vi "VI Tree.vi"   [LabVIEW 2020, in "Rohde&Schwarz CMXP Base.lvlib"]
doc: "This is the instrument driver for the Rohde&Schwarz CMX/CMP/PVT Base system. \n\nThe VI Tree displays all the user-callable VIs of the instrument driver in an organized table.\n\nFor detailed driver information including modification history, refer to the <B>rsvna.chm </B>file."
uses:
  <instrlib>/Rohde&Schwarz CMXP Base/Rohde&Schwarz CMXP Base.lvlib
panel:
  # "rsCmxpBase"
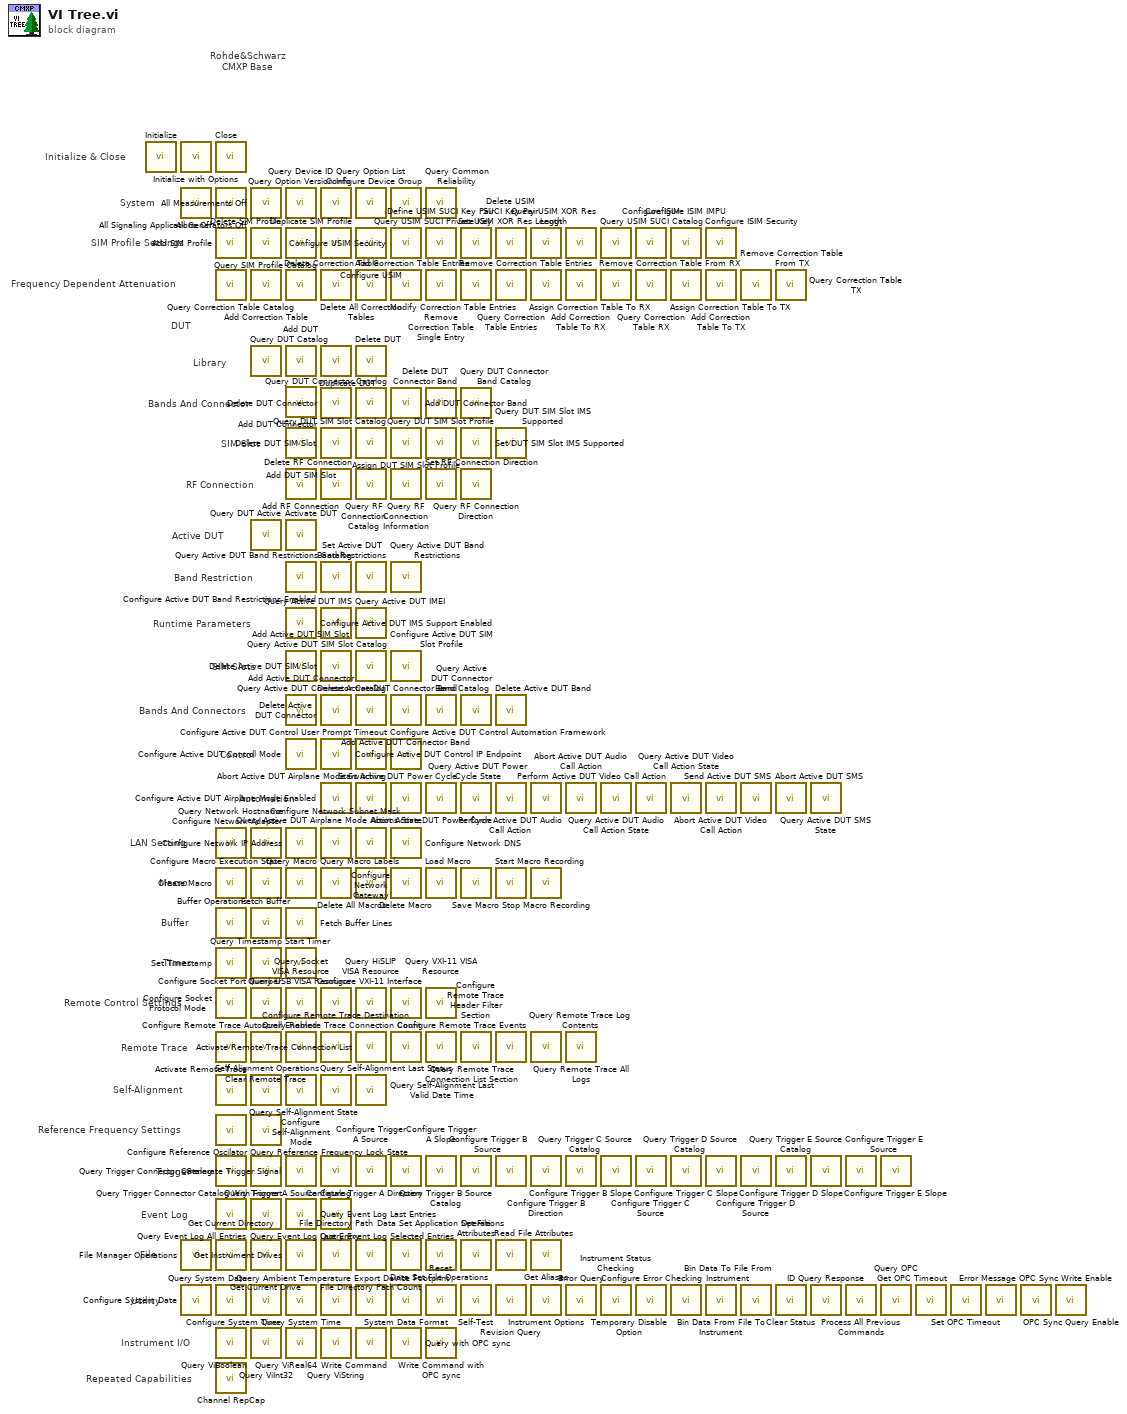
[diagram p0: block diagram]
diagram:
  # "Repeated Capabilities"
  # "Automation"
  # "Control"
  # "Bands And Connectors"
  # "SIM Slots"
  # "Runtime Parameters"
  # "Band Restriction"
  # "RF Connection"
  # "Active DUT"
  # "SIM Slot"
  # "Bands And Connector"
  # "Library"
  # "DUT"
  # "Frequency Dependent Attenuation"
  # "Remote Trace"
  # "Event Log"
  # "Trigger"
  # "File"
  # "Reference Frequency Settings"
  # "Self-Alignment"
  # "Remote Control Settings"
  # "Timer"
  # "Buffer"
  # "Macro"
  # "LAN Setting"
  # "SIM Profile Settings"
  # "System"
  # "Rohde&Schwarz \n    CMXP Base"
  # "Instrument I/O"
  # "Utility"
  # "Initialize & Close"
  n1 = call <instrlib>:"Initialize.vi"() -> ()  [unwired: 10 in, 2 out]
  n2 = call <instrlib>:"Initialize with Options.vi"() -> ()  [unwired: 10 in, 2 out]
  n3 = call <instrlib>:"All Signaling Applications Off.vi"() -> ()  [unwired: 10 in, 2 out]
  n4 = call <instrlib>:"File Manager Operations.vi"() -> ()  [unwired: 10 in, 2 out]
  n5 = call <instrlib>:"Configure System Date.vi"() -> ()  [unwired: 10 in, 2 out]
  n6 = call <instrlib>:"Close.vi"() -> ()  [unwired: 11 in, 1 out]
  n7 = call <instrlib>:"All Generators Off.vi"() -> ()  [unwired: 10 in, 2 out]
  n8 = call <instrlib>:"Add SIM Profile.vi"() -> ()  [unwired: 10 in, 2 out]
  n9 = call <instrlib>:"Query Correction Table Catalog.vi"() -> ()  [unwired: 9 in, 3 out]
  n10 = call <instrlib>:"Query Network Hostname.vi"() -> ()  [unwired: 9 in, 3 out]
  n11 = call <instrlib>:"Create Macro.vi"() -> ()  [unwired: 10 in, 2 out]
  n12 = call <instrlib>:"Buffer Operations.vi"() -> ()  [unwired: 10 in, 2 out]
  n13 = call <instrlib>:"Set Timestamp.vi"() -> ()  [unwired: 10 in, 2 out]
  n14 = call <instrlib>:"Configure Socket Protocol Mode.vi"() -> ()  [unwired: 10 in, 2 out]
  n15 = call <instrlib>:"Activate Remote Trace.vi"() -> ()  [unwired: 10 in, 2 out]
  n16 = call <instrlib>:"Self-Alignment Operations.vi"() -> ()  [unwired: 10 in, 2 out]
  n17 = call <instrlib>:"Configure Reference Oscilator.vi"() -> ()  [unwired: 10 in, 2 out]
  n18 = call <instrlib>:"Query Trigger Connector Catalog.vi"() -> ()  [unwired: 9 in, 3 out]
  n19 = call <instrlib>:"Query Event Log All Entries.vi"() -> ()  [unwired: 9 in, 3 out]
  n20 = call <instrlib>:"Get Current Directory.vi"() -> ()  [unwired: 9 in, 3 out]
  n21 = call <instrlib>:"Query System Date.vi"() -> ()  [unwired: 7 in, 5 out]
  n22 = call <instrlib>:"Query ViBoolean.vi"() -> ()  [unwired: 9 in, 3 out]
  n23 = call <instrlib>:"Channel RepCap.vi"() -> ()  [unwired: 1 in, 2 out]
  n24 = call <instrlib>:"All Measurements Off.vi"() -> ()  [unwired: 10 in, 2 out]
  n25 = call <instrlib>:"Delete SIM Profile.vi"() -> ()  [unwired: 10 in, 2 out]
  n26 = call <instrlib>:"Add Correction Table.vi"() -> ()  [unwired: 10 in, 2 out]
  n27 = call <instrlib>:"Query DUT Catalog.vi"() -> ()  [unwired: 9 in, 3 out]
  n28 = call <instrlib>:"Query DUT Active.vi"() -> ()  [unwired: 9 in, 3 out]
  n29 = call <instrlib>:"Configure Network Adapter.vi"() -> ()  [unwired: 10 in, 2 out]
  n30 = call <instrlib>:"Configure Macro Execution State.vi"() -> ()  [unwired: 10 in, 2 out]
  n31 = call <instrlib>:"Fetch Buffer.vi"() -> ()  [unwired: 9 in, 3 out]
  n32 = call <instrlib>:"Query Timestamp.vi"() -> ()  [unwired: 9 in, 3 out]
  n33 = call <instrlib>:"Configure Socket Port Number.vi"() -> ()  [unwired: 10 in, 2 out]
  n34 = call <instrlib>:"Clear Remote Trace.vi"() -> ()  [unwired: 10 in, 2 out]
  n35 = call <instrlib>:"Query Self-Alignment State.vi"() -> ()  [unwired: 9 in, 3 out]
  n36 = call <instrlib>:"Query Reference Frequency Lock State.vi"() -> ()  [unwired: 9 in, 3 out]
  n37 = call <instrlib>:"Query Trigger Connector Catalog With Format.vi"() -> ()  [unwired: 9 in, 3 out]
  n38 = call <instrlib>:"Query Event Log Last Entry.vi"() -> ()  [unwired: 7 in, 5 out]
  n39 = call <instrlib>:"Get Current Drive.vi"() -> ()  [unwired: 9 in, 3 out]
  n40 = call <instrlib>:"Configure System Time.vi"() -> ()  [unwired: 10 in, 2 out]
  n41 = call <instrlib>:"Query ViInt32.vi"() -> ()  [unwired: 9 in, 3 out]
  n42 = call <instrlib>:"Query Device ID.vi"() -> ()  [unwired: 9 in, 3 out]
  n43 = call <instrlib>:"Query SIM Profile Catalog.vi"() -> ()  [unwired: 9 in, 3 out]
  n44 = call <instrlib>:"Delete Correction Table.vi"() -> ()  [unwired: 10 in, 2 out]
  n45 = call <instrlib>:"Add DUT.vi"() -> ()  [unwired: 10 in, 2 out]
  n46 = call <instrlib>:"Add DUT Connector.vi"() -> ()  [unwired: 10 in, 2 out]
  n47 = call <instrlib>:"Add DUT SIM Slot.vi"() -> ()  [unwired: 10 in, 2 out]
  n48 = call <instrlib>:"Add RF Connection.vi"() -> ()  [unwired: 10 in, 2 out]
  n49 = call <instrlib>:"Activate DUT.vi"() -> ()  [unwired: 10 in, 2 out]
  n50 = call <instrlib>:"Configure Active DUT Band Restrictions Enabled.vi"() -> ()  [unwired: 10 in, 2 out]
  n51 = call <instrlib>:"Configure Active DUT IMS Support Enabled.vi"() -> ()  [unwired: 10 in, 2 out]
  n52 = call <instrlib>:"Add Active DUT SIM Slot.vi"() -> ()  [unwired: 10 in, 2 out]
  n53 = call <instrlib>:"Add Active DUT Connector.vi"() -> ()  [unwired: 10 in, 2 out]
  n54 = call <instrlib>:"Configure Active DUT Control Mode.vi"() -> ()  [unwired: 10 in, 2 out]
  n55 = call <instrlib>:"Configure Network IP Address.vi"() -> ()  [unwired: 10 in, 2 out]
  n56 = call <instrlib>:"Query Macro.vi"() -> ()  [unwired: 9 in, 3 out]
  n57 = call <instrlib>:"Fetch Buffer Lines.vi"() -> ()  [unwired: 9 in, 3 out]
  n58 = call <instrlib>:"Start Timer.vi"() -> ()  [unwired: 10 in, 2 out]
  n59 = call <instrlib>:"Query Socket VISA Resource.vi"() -> ()  [unwired: 9 in, 3 out]
  n60 = call <instrlib>:"Configure Remote Trace Autoscroll Enabled.vi"() -> ()  [unwired: 10 in, 2 out]
  n61 = call <instrlib>:"Configure Self-Alignment Mode.vi"() -> ()  [unwired: 10 in, 2 out]
  n62 = call <instrlib>:"Generate Trigger Signal.vi"() -> ()  [unwired: 10 in, 2 out]
  n63 = call <instrlib>:"Query Event Log Last Entries.vi"() -> ()  [unwired: 10 in, 2 out]
  n64 = call <instrlib>:"Get Instrument Drives.vi"() -> ()  [unwired: 9 in, 3 out]
  n65 = call <instrlib>:"Query System Time.vi"() -> ()  [unwired: 7 in, 5 out]
  n66 = call <instrlib>:"Query ViReal64.vi"() -> ()  [unwired: 9 in, 3 out]
  n67 = call <instrlib>:"Query Option Version Info.vi"() -> ()  [unwired: 9 in, 3 out]
  n68 = call <instrlib>:"Duplicate SIM Profile.vi"() -> ()  [unwired: 10 in, 2 out]
  n69 = call <instrlib>:"Delete All Correction Tables.vi"() -> ()  [unwired: 10 in, 2 out]
  n70 = call <instrlib>:"Duplicate DUT.vi"() -> ()  [unwired: 10 in, 2 out]
  n71 = call <instrlib>:"Delete DUT Connector.vi"() -> ()  [unwired: 10 in, 2 out]
  n72 = call <instrlib>:"Delete DUT SIM Slot.vi"() -> ()  [unwired: 10 in, 2 out]
  n73 = call <instrlib>:"Delete RF Connection.vi"() -> ()  [unwired: 10 in, 2 out]
  n74 = call <instrlib>:"Query Active DUT Band Restrictions Catalog.vi"() -> ()  [unwired: 9 in, 3 out]
  n75 = call <instrlib>:"Query Active DUT IMS.vi"() -> ()  [unwired: 9 in, 3 out]
  n76 = call <instrlib>:"Delete Active DUT SIM Slot.vi"() -> ()  [unwired: 10 in, 2 out]
  n77 = call <instrlib>:"Delete Active DUT Connector.vi"() -> ()  [unwired: 10 in, 2 out]
  n78 = call <instrlib>:"Configure Active DUT Control IP Endpoint.vi"() -> ()  [unwired: 10 in, 2 out]
  n79 = call <instrlib>:"Configure Active DUT Airplane Mode Enabled.vi"() -> ()  [unwired: 10 in, 2 out]
  n80 = call <instrlib>:"Configure Network Subnet Mask.vi"() -> ()  [unwired: 10 in, 2 out]
  n81 = call <instrlib>:"Query Macro Labels.vi"() -> ()  [unwired: 9 in, 3 out]
  n82 = call <instrlib>:"Query USB VISA Resource.vi"() -> ()  [unwired: 9 in, 3 out]
  n83 = call <instrlib>:"Configure Remote Trace Destination.vi"() -> ()  [unwired: 10 in, 2 out]
  n84 = call <instrlib>:"Query Self-Alignment Last Status.vi"() -> ()  [unwired: 8 in, 4 out]
  n85 = call <instrlib>:"Query Trigger A Source Catalog.vi"() -> ()  [unwired: 9 in, 3 out]
  n86 = call <instrlib>:"Query Event Log Selected Entries.vi"() -> ()  [unwired: 10 in, 2 out]
  n87 = call <instrlib>:"File Directory Path.vi"() -> ()  [unwired: 9 in, 3 out]
  n88 = call <instrlib>:"Query Ambient Temperature.vi"() -> ()  [unwired: 7 in, 5 out]
  n89 = call <instrlib>:"Query ViString.vi"() -> ()  [unwired: 9 in, 3 out]
  n90 = call <instrlib>:"Query Option List.vi"() -> ()  [unwired: 9 in, 3 out]
  n91 = call <instrlib>:"Configure USIM.vi"() -> ()  [unwired: 10 in, 2 out]
  n92 = call <instrlib>:"Add Correction Table Entries.vi"() -> ()  [unwired: 10 in, 2 out]
  n93 = call <instrlib>:"Delete DUT.vi"() -> ()  [unwired: 10 in, 2 out]
  n94 = call <instrlib>:"Query DUT Connector Catalog.vi"() -> ()  [unwired: 9 in, 3 out]
  n95 = call <instrlib>:"Query DUT SIM Slot Catalog.vi"() -> ()  [unwired: 9 in, 3 out]
  n96 = call <instrlib>:"Query RF Connection Catalog.vi"() -> ()  [unwired: 9 in, 3 out]
  n97 = call <instrlib>:"Set Active DUT Band Restrictions.vi"() -> ()  [unwired: 10 in, 2 out]
  n98 = call <instrlib>:"Query Active DUT IMEI.vi"() -> ()  [unwired: 9 in, 3 out]
  n99 = call <instrlib>:"Query Active DUT SIM Slot Catalog.vi"() -> ()  [unwired: 9 in, 3 out]
  n100 = call <instrlib>:"Query Active DUT Connector Catalog.vi"() -> ()  [unwired: 9 in, 3 out]
  n101 = call <instrlib>:"Configure Active DUT Control User Prompt Timeout.vi"() -> ()  [unwired: 10 in, 2 out]
  n102 = call <instrlib>:"Abort Active DUT Airplane Mode Switching.vi"() -> ()  [unwired: 10 in, 2 out]
  n103 = call <instrlib>:"Configure Network Gateway.vi"() -> ()  [unwired: 10 in, 2 out]
  n104 = call <instrlib>:"Delete All Macros.vi"() -> ()  [unwired: 10 in, 2 out]
  n105 = call <instrlib>:"Query HiSLIP VISA Resource.vi"() -> ()  [unwired: 9 in, 3 out]
  n106 = call <instrlib>:"Activate Remote Trace Connection List.vi"() -> ()  [unwired: 10 in, 2 out]
  n107 = call <instrlib>:"Query Self-Alignment Last Valid Date Time.vi"() -> ()  [unwired: 6 in, 6 out]
  n108 = call <instrlib>:"Configure Trigger A Source.vi"() -> ()  [unwired: 10 in, 2 out]
  n109 = call <instrlib>:"File Directory Path Count.vi"() -> ()  [unwired: 9 in, 3 out]
  n110 = call <instrlib>:"Export Device Footprint.vi"() -> ()  [unwired: 10 in, 2 out]
  n111 = call <instrlib>:"Write Command.vi"() -> ()  [unwired: 10 in, 2 out]
  n112 = call <instrlib>:"Configure Device Group.vi"() -> ()  [unwired: 10 in, 2 out]
  n113 = call <instrlib>:"Configure USIM Security.vi"() -> ()  [unwired: 14 in, 2 out]
  n114 = call <instrlib>:"Modify Correction Table Entries.vi"() -> ()  [unwired: 10 in, 2 out]
  n115 = call <instrlib>:"Add DUT Connector Band.vi"() -> ()  [unwired: 10 in, 2 out]
  n116 = call <instrlib>:"Assign DUT SIM Slot Profile.vi"() -> ()  [unwired: 10 in, 2 out]
  n117 = call <instrlib>:"Query RF Connection Information.vi"() -> ()  [unwired: 9 in, 3 out]
  n118 = call <instrlib>:"Query Active DUT Band Restrictions.vi"() -> ()  [unwired: 8 in, 4 out]
  n119 = call <instrlib>:"Configure Active DUT SIM Slot Profile.vi"() -> ()  [unwired: 10 in, 2 out]
  n120 = call <instrlib>:"Add Active DUT Connector Band.vi"() -> ()  [unwired: 10 in, 2 out]
  n121 = call <instrlib>:"Configure Active DUT Control Automation Framework.vi"() -> ()  [unwired: 10 in, 2 out]
  n122 = call <instrlib>:"Query Active DUT Airplane Mode Actions State.vi"() -> ()  [unwired: 8 in, 4 out]
  n123 = call <instrlib>:"Configure Network DNS.vi"() -> ()  [unwired: 10 in, 2 out]
  n124 = call <instrlib>:"Delete Macro.vi"() -> ()  [unwired: 10 in, 2 out]
  n125 = call <instrlib>:"Configure VXI-11 Interface.vi"() -> ()  [unwired: 10 in, 2 out]
  n126 = call <instrlib>:"Query Remote Trace Connection Count.vi"() -> ()  [unwired: 8 in, 4 out]
  n127 = call <instrlib>:"Configure Trigger A Direction.vi"() -> ()  [unwired: 10 in, 2 out]
  n128 = call <instrlib>:"Data Set File Operations.vi"() -> ()  [unwired: 10 in, 2 out]
  n129 = call <instrlib>:"System Data Format.vi"() -> ()  [unwired: 10 in, 2 out]
  n130 = call <instrlib>:"Query with OPC sync.vi"() -> ()  [unwired: 9 in, 3 out]
  n131 = call <instrlib>:"Query Common Reliability.vi"() -> ()  [unwired: 9 in, 3 out]
  n132 = call <instrlib>:"Define USIM SUCI Key Pair.vi"() -> ()  [unwired: 10 in, 2 out]
  n133 = call <instrlib>:"Remove Correction Table Single Entry.vi"() -> ()  [unwired: 10 in, 2 out]
  n134 = call <instrlib>:"Delete DUT Connector Band.vi"() -> ()  [unwired: 10 in, 2 out]
  n135 = call <instrlib>:"Query DUT SIM Slot Profile.vi"() -> ()  [unwired: 9 in, 3 out]
  n136 = call <instrlib>:"Set RF Connection Direction.vi"() -> ()  [unwired: 10 in, 2 out]
  n137 = call <instrlib>:"Delete Active DUT Connector Band.vi"() -> ()  [unwired: 10 in, 2 out]
  n138 = call <instrlib>:"Start Active DUT Power Cycle.vi"() -> ()  [unwired: 10 in, 2 out]
  n139 = call <instrlib>:"Load Macro.vi"() -> ()  [unwired: 10 in, 2 out]
  n140 = call <instrlib>:"Query VXI-11 VISA Resource.vi"() -> ()  [unwired: 9 in, 3 out]
  n141 = call <instrlib>:"Query Remote Trace Connection List Section.vi"() -> ()  [unwired: 9 in, 3 out]
  n142 = call <instrlib>:"Configure Trigger A Slope.vi"() -> ()  [unwired: 10 in, 2 out]
  n143 = call <instrlib>:"Data Set Application Operations.vi"() -> ()  [unwired: 10 in, 2 out]
  n144 = call <instrlib>:"Reset.vi"() -> ()  [unwired: 10 in, 2 out]
  n145 = call <instrlib>:"Write Command with OPC sync.vi"() -> ()  [unwired: 10 in, 2 out]
  n146 = call <instrlib>:"Query USIM SUCI Private Key.vi"() -> ()  [unwired: 9 in, 3 out]
  n147 = call <instrlib>:"Remove Correction Table Entries.vi"() -> ()  [unwired: 10 in, 2 out]
  n148 = call <instrlib>:"Query DUT Connector Band Catalog.vi"() -> ()  [unwired: 9 in, 3 out]
  n149 = call <instrlib>:"Set DUT SIM Slot IMS Supported.vi"() -> ()  [unwired: 10 in, 2 out]
  n150 = call <instrlib>:"Query RF Connection Direction.vi"() -> ()  [unwired: 10 in, 2 out]
  n151 = call <instrlib>:"Query Active DUT Connector Band Catalog.vi"() -> ()  [unwired: 9 in, 3 out]
  n152 = call <instrlib>:"Abort Active DUT Power Cycle.vi"() -> ()  [unwired: 10 in, 2 out]
  n153 = call <instrlib>:"Save Macro.vi"() -> ()  [unwired: 10 in, 2 out]
  n154 = call <instrlib>:"Configure Remote Trace Header Filter Section.vi"() -> ()  [unwired: 10 in, 2 out]
  n155 = call <instrlib>:"Query Trigger B Source Catalog.vi"() -> ()  [unwired: 9 in, 3 out]
  n156 = call <instrlib>:"Set File Attributes.vi"() -> ()  [unwired: 10 in, 2 out]
  n157 = call <instrlib>:"Self-Test.vi"() -> ()  [unwired: 8 in, 4 out]
  n158 = call <instrlib>:"Delete USIM SUCI Key Pair.vi"() -> ()  [unwired: 10 in, 2 out]
  n159 = call <instrlib>:"Query Correction Table Entries.vi"() -> ()  [unwired: 9 in, 3 out]
  n160 = call <instrlib>:"Query DUT SIM Slot IMS Supported.vi"() -> ()  [unwired: 9 in, 3 out]
  n161 = call <instrlib>:"Delete Active DUT Band.vi"() -> ()  [unwired: 10 in, 2 out]
  n162 = call <instrlib>:"Query Active DUT Power Cycle State.vi"() -> ()  [unwired: 9 in, 3 out]
  n163 = call <instrlib>:"Start Macro Recording.vi"() -> ()  [unwired: 10 in, 2 out]
  n164 = call <instrlib>:"Configure Remote Trace Events.vi"() -> ()  [unwired: 10 in, 2 out]
  n165 = call <instrlib>:"Configure Trigger B Source.vi"() -> ()  [unwired: 10 in, 2 out]
  n166 = call <instrlib>:"Read File Attributes.vi"() -> ()  [unwired: 9 in, 3 out]
  n167 = call <instrlib>:"Revision Query.vi"() -> ()  [unwired: 8 in, 4 out]
  n168 = call <instrlib>:"Set USIM XOR Res Length.vi"() -> ()  [unwired: 10 in, 2 out]
  n169 = call <instrlib>:"Assign Correction Table To RX.vi"() -> ()  [unwired: 10 in, 2 out]
  n170 = call <instrlib>:"Perform Active DUT Audio Call Action.vi"() -> ()  [unwired: 10 in, 2 out]
  n171 = call <instrlib>:"Stop Macro Recording.vi"() -> ()  [unwired: 10 in, 2 out]
  n172 = call <instrlib>:"Query Remote Trace Log Contents.vi"() -> ()  [unwired: 9 in, 3 out]
  n173 = call <instrlib>:"Configure Trigger B Direction.vi"() -> ()  [unwired: 10 in, 2 out]
  n174 = call <instrlib>:"Get Aliases.vi"() -> ()  [unwired: 9 in, 3 out]
  n175 = call <instrlib>:"Instrument Options.vi"() -> ()  [unwired: 9 in, 3 out]
  n176 = call <instrlib>:"Query USIM XOR Res Length.vi"() -> ()  [unwired: 9 in, 3 out]
  n177 = call <instrlib>:"Add Correction Table To RX.vi"() -> ()  [unwired: 10 in, 2 out]
  n178 = call <instrlib>:"Abort Active DUT Audio Call Action.vi"() -> ()  [unwired: 10 in, 2 out]
  n179 = call <instrlib>:"Query Remote Trace All Logs.vi"() -> ()  [unwired: 9 in, 3 out]
  n180 = call <instrlib>:"Configure Trigger B Slope.vi"() -> ()  [unwired: 10 in, 2 out]
  n181 = call <instrlib>:"Error Query.vi"() -> ()  [unwired: 8 in, 4 out]
  n182 = call <instrlib>:"Query USIM SUCI Catalog.vi"() -> ()  [unwired: 9 in, 3 out]
  n183 = call <instrlib>:"Remove Correction Table From RX.vi"() -> ()  [unwired: 10 in, 2 out]
  n184 = call <instrlib>:"Query Active DUT Audio Call Action State.vi"() -> ()  [unwired: 6 in, 6 out]
  n185 = call <instrlib>:"Query Trigger C Source Catalog.vi"() -> ()  [unwired: 9 in, 3 out]
  n186 = call <instrlib>:"Instrument Status Checking.vi"() -> ()  [unwired: 10 in, 2 out]
  n187 = call <instrlib>:"Configure ISIM.vi"() -> ()  [unwired: 10 in, 2 out]
  n188 = call <instrlib>:"Query Correction Table RX.vi"() -> ()  [unwired: 9 in, 3 out]
  n189 = call <instrlib>:"Perform Active DUT Video Call Action.vi"() -> ()  [unwired: 10 in, 2 out]
  n190 = call <instrlib>:"Configure Trigger C Source.vi"() -> ()  [unwired: 10 in, 2 out]
  n191 = call <instrlib>:"Temporary Disable Option.vi"() -> ()  [unwired: 10 in, 2 out]
  n192 = call <instrlib>:"Configure ISIM IMPU.vi"() -> ()  [unwired: 10 in, 2 out]
  n193 = call <instrlib>:"Assign Correction Table To TX.vi"() -> ()  [unwired: 10 in, 2 out]
  n194 = call <instrlib>:"Query Active DUT Video Call Action State.vi"() -> ()  [unwired: 6 in, 6 out]
  n195 = call <instrlib>:"Configure Trigger C Slope.vi"() -> ()  [unwired: 10 in, 2 out]
  n196 = call <instrlib>:"Configure Error Checking.vi"() -> ()  [unwired: 10 in, 2 out]
  n197 = call <instrlib>:"Configure ISIM Security.vi"() -> ()  [unwired: 14 in, 2 out]
  n198 = call <instrlib>:"Add Correction Table To TX.vi"() -> ()  [unwired: 10 in, 2 out]
  n199 = call <instrlib>:"Abort Active DUT Video Call Action.vi"() -> ()  [unwired: 10 in, 2 out]
  n200 = call <instrlib>:"Query Trigger D Source Catalog.vi"() -> ()  [unwired: 9 in, 3 out]
  n201 = call <instrlib>:"Bin Data From File To Instrument.vi"() -> ()  [unwired: 10 in, 2 out]
  n202 = call <instrlib>:"Remove Correction Table From TX.vi"() -> ()  [unwired: 10 in, 2 out]
  n203 = call <instrlib>:"Send Active DUT SMS.vi"() -> ()  [unwired: 10 in, 2 out]
  n204 = call <instrlib>:"Configure Trigger D Source.vi"() -> ()  [unwired: 10 in, 2 out]
  n205 = call <instrlib>:"Bin Data To File From Instrument.vi"() -> ()  [unwired: 10 in, 2 out]
  n206 = call <instrlib>:"Query Correction Table TX.vi"() -> ()  [unwired: 9 in, 3 out]
  n207 = call <instrlib>:"Abort Active DUT SMS.vi"() -> ()  [unwired: 10 in, 2 out]
  n208 = call <instrlib>:"Configure Trigger D Slope.vi"() -> ()  [unwired: 10 in, 2 out]
  n209 = call <instrlib>:"Clear Status.vi"() -> ()  [unwired: 10 in, 2 out]
  n210 = call <instrlib>:"Query Active DUT SMS State.vi"() -> ()  [unwired: 9 in, 3 out]
  n211 = call <instrlib>:"Query Trigger E Source Catalog.vi"() -> ()  [unwired: 9 in, 3 out]
  n212 = call <instrlib>:"ID Query Response.vi"() -> ()  [unwired: 9 in, 3 out]
  n213 = call <instrlib>:"Configure Trigger E Source.vi"() -> ()  [unwired: 10 in, 2 out]
  n214 = call <instrlib>:"Process All Previous Commands.vi"() -> ()  [unwired: 10 in, 2 out]
  n215 = call <instrlib>:"Configure Trigger E Slope.vi"() -> ()  [unwired: 10 in, 2 out]
  n216 = call <instrlib>:"Query OPC.vi"() -> ()  [unwired: 9 in, 3 out]
  n217 = call <instrlib>:"Get OPC Timeout.vi"() -> ()  [unwired: 9 in, 3 out]
  n218 = call <instrlib>:"Set OPC Timeout.vi"() -> ()  [unwired: 10 in, 2 out]
  n219 = call <instrlib>:"Error Message.vi"() -> ()  [unwired: 7 in, 5 out]
  n220 = call <instrlib>:"OPC Sync Write Enable.vi"() -> ()  [unwired: 10 in, 2 out]
  n221 = call <instrlib>:"OPC Sync Query Enable.vi"() -> ()  [unwired: 10 in, 2 out]
